vi "Test Cannot Get VI Ref Before Start.vi"(8 "error in (no error)":errorcluster, 11 "View Test In":refnum<class "View Dev Test.lvclass">) -> (0 "error out":errorcluster, 3 "View Test Out":refnum<class "View Dev Test.lvclass">)   [LabVIEW 2020, in "View Dev Test.lvclass"]
uses:
  View Dev Test.lvclass
  C:/Program Files (x86)/National Instruments/LabVIEW 2020/vi.lib/Astemes/LUnit/Test Case.lvclass
  source/Framework/Process/Process.lvclass/Process.ctl
  source/Framework/Synchronous Request Callback/Synchronous Request Callback.lvclass/Synchronous Request Callback.ctl
  <vilib>/Astemes/LUnit/Test Case.lvclass/Test Case.ctl
  source/Framework/Process/Protected/Messaging/Request Message.vi
  source/Framework/Process/Public/Lifecycle/Get Lifecycle State.vi
  <vilib>/Astemes/LUnit/Append Fail Result.vi
  <vilib>/Astemes/LUnit/Append Pass Result.vi
  source/Framework/Process/Private/SubVIs/Handle Debug Data.vi
  source/Framework/Process/Private/SubVIs/Enqueue Request Message.vi
  source/Framework/Synchronous Request Callback/Create.vi
  <vilib>/Utility/error.llb/Clear Errors.vi
  source/Framework/Logging/Log Debug.vi
  <vilib>/AdvancedString/1D String Array to Delimited String.vi
  <vilib>/Utility/High Resolution Relative Seconds.vi
  source/Framework/View/View.lvclass
  C:/git/astemes-triarc-framework/source/Framework/Process/Process.lvclass
  source/Framework/Synchronous Request Callback/Synchronous Request Callback.lvclass
  C:/git/astemes-triarc-framework/source/Framework/Callback/Callback.lvclass
  source/Framework/Process/Process.lvclass
  C:/git/astemes-triarc-framework/source/Framework/Logging/Logging.lvclass
  <vilib>/Utility/error.llb/Error Cluster From Error Code.vi
  source/Framework/Process/Public/Read Name.vi
  source/Framework/Process/Private/SubVIs/Wait for Response Message.vi
  source/Framework/Callback/Callback.lvclass
  source/Framework/Logging/Logging.lvclass
  View Dev Test.lvclass/View Dev Test.ctl
  <vilib>/Astemes/LUnit/Test Case.lvclass
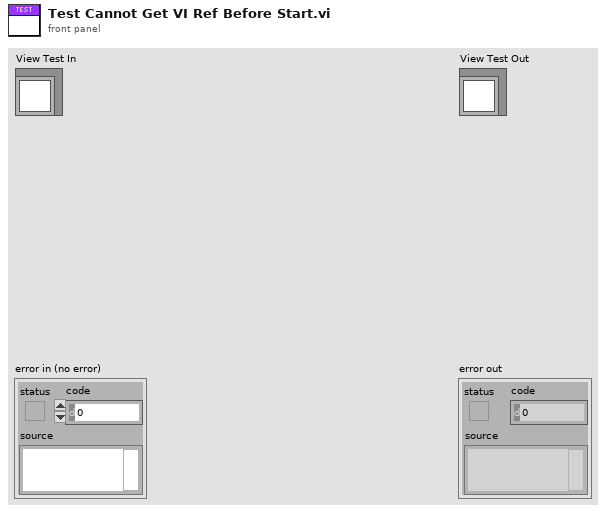
[diagram p1: front panel]
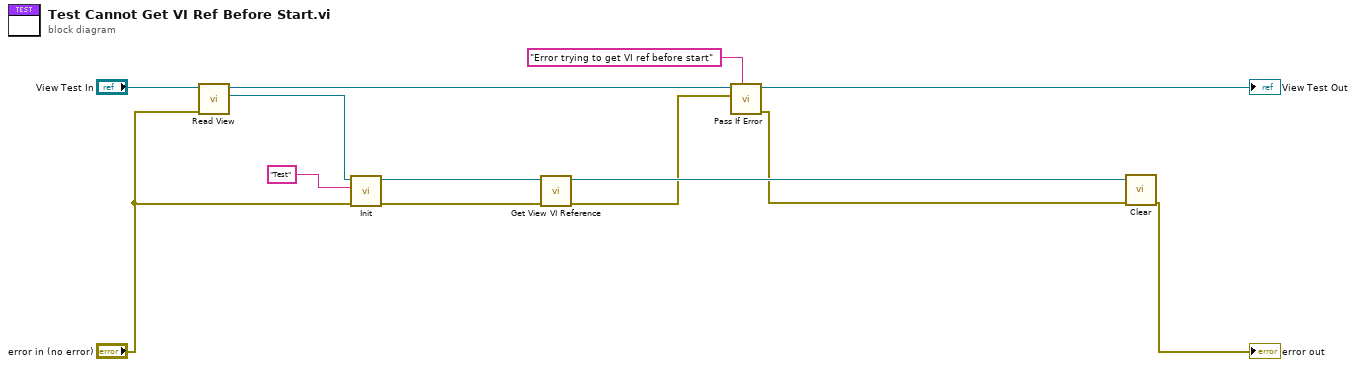
[diagram p0: block diagram]
diagram:
  n1 = call "Read View.vi"("error in (no error)"="error in (no error)", "View Test In"="View Test In") -> ("View"=w12:refnum<class "View.lvclass">, "View Test Out"=w13:refnum<class "View Dev Test.lvclass">)  [unwired: 7 in, 1 out]
  n2 = call-dynamic "Init.vi"("error in (no error)"="error in (no error)", "Name"="Test", "View In"=w12) -> ("error out"=w6:errorcluster, "View Out"=w7:refnum<class "View.lvclass">)  [unwired: 7 in]
  n3 = call "Get View VI Reference.vi"("error in (no error)"=w6, "View In"=w7) -> ("error out"=w3:errorcluster, "View Out"=w5:refnum<class "View.lvclass">)  [unwired: 7 in, 1 out]
  n4 = call <vilib>:"Pass If Error.vi"("Description"="Error trying to get VI ref before start", "Assert error"=w3, "LUnit Test Case In"=w13) -> ("error out"=w1:errorcluster, "LUnit Test Case Out"=→"View Test Out":refnum<class "View Dev Test.lvclass">)  [unwired: 7 in]
  n5 = call-dynamic "Clear.vi"("error in (no error)"=w1, "View In"=w5) -> ("error out"=→"error out":errorcluster)  [unwired: 9 in]
